vi "GetTagFromPath.vi"(0 "Tree Ref In":refnum<vi>, 5 "Hierarchical Path":string, 11 "Error In":errorcluster) -> (4 "Tree Ref Out":refnum<vi>, 6 "Item Tag":string, 8 "Item Found?":bool, 15 "Error Out":errorcluster)   [LabVIEW 2016, in "Drona.lvlib"]
doc: "Get the item tag of tree control from the input hierarchical path"
uses:
  Drona.lvlib
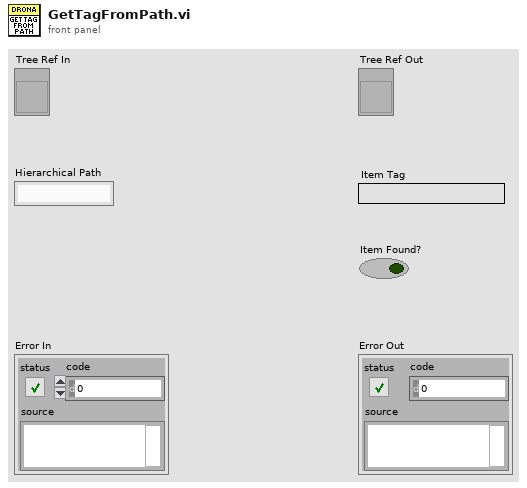
[diagram p1: front panel]
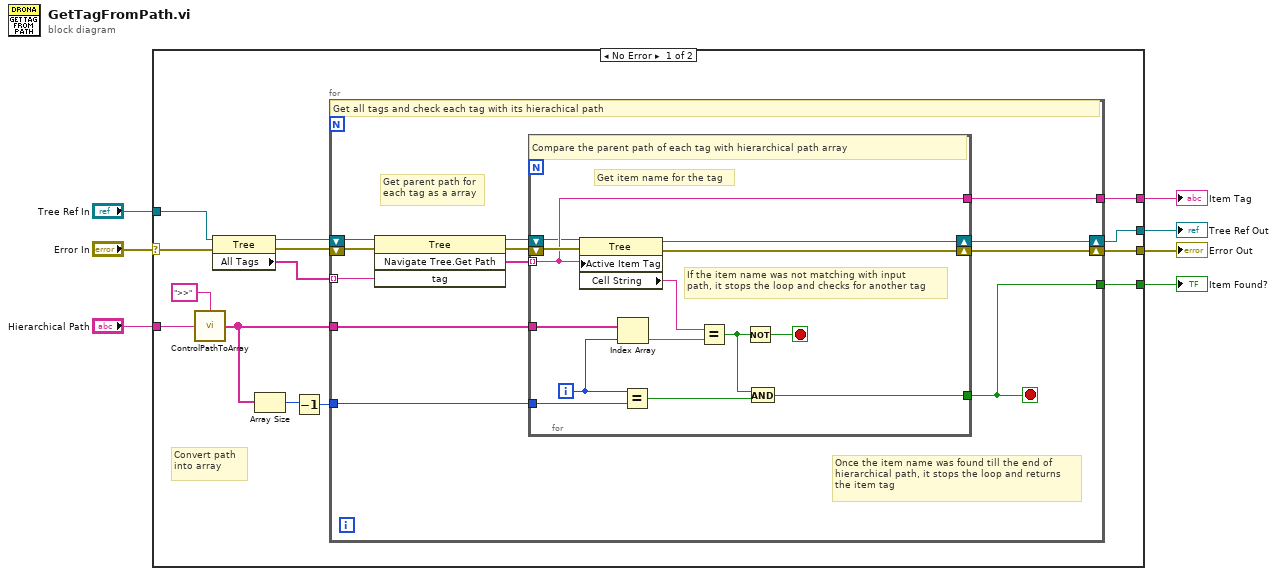
[diagram p0: block diagram]
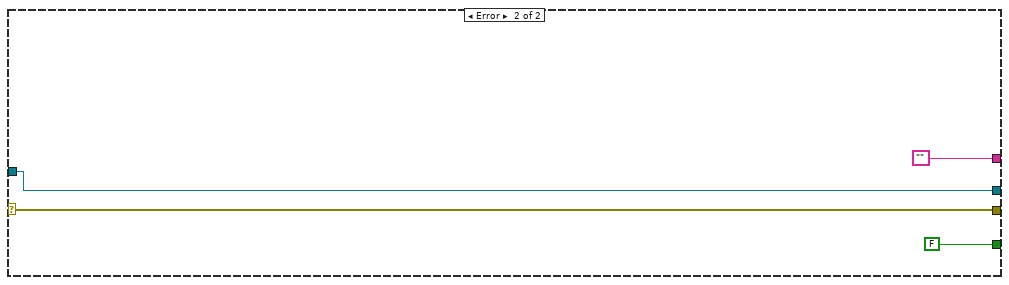
[diagram p2: hidden frame]
diagram:
  n1 = case shown="No Error" "Error In" {
    selector: "Error In" -> [w14 w50]
    tunnel: "Tree Ref In" -> [w13 w51]
    tunnel: "Hierarchical Path" -> [w12 _]
    tunnel: [w11 ""] -> w4
    tunnel: [w10 w51] -> w3
    tunnel: [w9 w50] -> w2
    tunnel: [w8 FALSE] -> w1
    frame No Error {
      # "Convert path \ninto array"
      n2 = call "ControlPathToArray.vi"("Control Name"=w12, "delimiter (>>)"=">>") -> ("Control Path"=w16:string[])
      n3 = property class="Tree"(reference=w13, error in=w14) -> (reference out=w20:refnum<vi>, error out=w21:errorcluster, "All Tags"=w19:string[])
      n4 = Array Size(array=w16) -> (size(s)=w17:i32)
      n5 = Decrement(x=w17) -> (x-1=w15:i32)
      n6 = for {
        tunnel: w19 -> [w33] mode=indexing
        tunnel: w16 -> [w29]
        tunnel: w15 -> [w28]
        shift-right: [w27] -> w9
        shift-left: w21 -> [w32]
        tunnel: [w26] -> w11
        shift-right: [w23] -> w10
        shift-left: w20 -> [w25]
        tunnel: [w22] -> w8
        stop <- w22 stop-if-true
        # "Once the item name was found till the end of \nhierarchical path, it stops the loop and returns \nthe item tag"
        # "Get parent path for\neach tag as a array"
        # "Get all tags and check each tag with its hierachical path"
        n7 = invoke class="Tree" method="Navigate Tree.Get Path"(reference=w25, error in=w32, "tag"=w33) -> (reference out=w24:refnum<vi>, error out=w31:errorcluster, "Navigate Tree:Get Path"=w30:string[])  [unwired: 1 in, 1 out]
        n8 = for {
          tunnel: w30 -> [w36] mode=indexing
          tunnel: w29 -> [w46]
          tunnel: w28 -> [w43]
          tunnel: [w39] -> w22
          shift-right: [w37] -> w27
          shift-left: w31 -> [w47]
          tunnel: [w36] -> w26
          shift-right: [w34] -> w23
          shift-left: w24 -> [w35]
          i -> [w42]
          stop <- w38 stop-if-true
          # "Get item name for the tag"
          # "If the item name was not matching with input \npath, it stops the loop and checks for another tag"
          # "Compare the parent path of each tag with hierarchical path array"
          n9 = property class="Tree"(reference=w35, error in=w47, "Active Item Tag"=w36) -> (reference out=w34:refnum<vi>, error out=w37:errorcluster, "Cell String"=w45:string)
          n10 = Index Array(array=w46, index=w42) -> (element=w44:string)
          n11 = Equal?(x=w42, y=w43) -> (x = y?=w40:bool)
          n12 = Equal?(x=w45, y=w44) -> (x = y?=w41:bool)
          n13 = Not(x=w41) -> (.not. x?=w38:bool)
          n14 = And(x=w41, y=w40) -> (x .and. y?=w39:bool)
        }
      }
    }
    frame Error {
    }
  }
  "Item Tag" <- w4
  "Tree Ref Out" <- w3
  "Error Out" <- w2
  "Item Found?" <- w1
